vi "Module Did Init.vi"(6 "This VI":refnum<vi>, 8 "error in":errorcluster, 9 "Initialized?":bool, 10 "Origin":string, 11 "Module ID":i32=-1) -> (0 "error out":errorcluster)   [LabVIEW 2025, in "Test Unit.lvlib"]
doc: "Send the Module Did Init event to any VI registered to listen to this module's broadcast events.\n_____\nBased on DQMH Project Template 7.0.1.1316."
uses:
  Test Unit.lvlib
  Did Init Argument--cluster.ctl
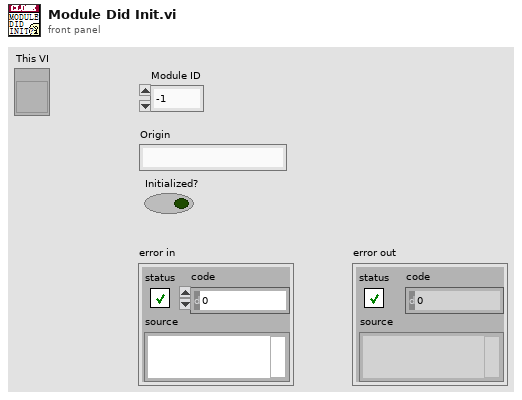
[diagram p1: front panel]
types:
  T1 = typedef "Test Unit.lvlib/Did Init Argument--cluster.ctl" = cluster{"Init?":bool, "Info":string, "Module ID":i32, "This VI":refnum<vi>}
  T2 = typedef "Test Unit.lvlib/Broadcast Events--cluster.ctl" = cluster{"Module Did Init":refnum<user-event>, "Status Updated":refnum<user-event>, "Error Reported":refnum<user-event>, "Module Did Stop":refnum<user-event>, "Update Module Execution Status":refnum<user-event>}
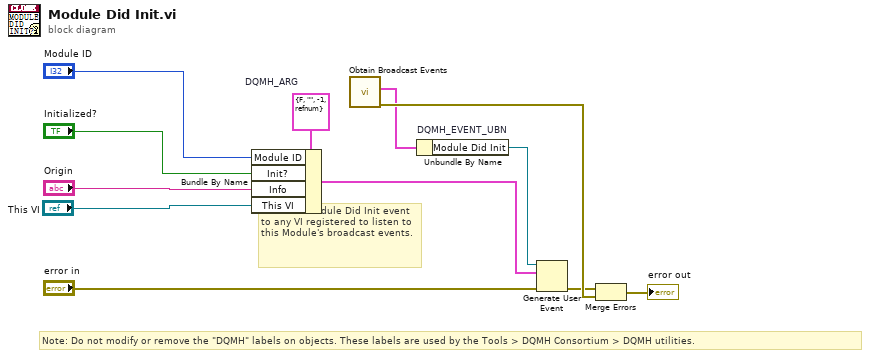
[diagram p0: block diagram]
diagram:
  w4 = T1 {"Init?"=FALSE, "Info"="", "Module ID"=-1, "This VI"=refnum}  # DQMH_ARG
  # "Note: Do not modify or remove the \"DQMH\" labels on objects. These labels are used by the Tools > DQMH Consortium > DQMH utilities."
  # "Send the Module Did Init event to any VI registered to listen to this Module's broadcast events."
  n1 = Bundle By Name(cluster=w4, "Module ID"="Module ID", "Init?"="Initialized?", "Info"="Origin", "This VI"="This VI") -> (w3:T1)
  n2 = call "Obtain Broadcast Events.vi"() -> ("error out"=w8:errorcluster, "Test Unit Broadcast Events"=w6:T2)  [unwired: 10 in]
  n3 = Unbundle By Name "DQMH_EVENT_UBN"(w6) -> ("Module Did Init"=w5:refnum<user-event>)
  n4 = Generate User Event(user event=w5, event data cluster=w3, error in="error in") -> (error out=w7:errorcluster)  [unwired: 1 in, 1 out]
  n5 = Merge Errors(w7, w8) -> (→"error out":errorcluster)
